vi "AI-Measure.vi"() -> ()   [LabVIEW 2016]
uses:
  <vilib>/DAQmx/read.llb/DAQmx Read (Analog Wfm 1Chan NSamp).vi
  <vilib>/DAQmx/miscellaneous.llb/DAQmx Fill In Error Info.vi
  <vilib>/Waveform/WDTFileIO.llb/Export Waveforms To Spreadsheet File (1D).vi
  <vilib>/Analysis/NI_AALBase.lvlib
  <vilib>/ptbypt/NI_PtbyPt.lvlib
panel:
  out "Signal Output":waveform(dbl)(graph)
  in  "file path (dialog if empty)":path
  out "Histogram Graph":T1(graph)
  out "Convergence of Standard Deviation":dbl[](graph)
  in  "Sample Time (s)":dbl=-1.0
  out "Convergence of Mean":dbl[](graph)
  out "standard deviation":dbl format="%0.2f"
  out "mean":dbl format="%0.2f"
  out "size(s)":i32
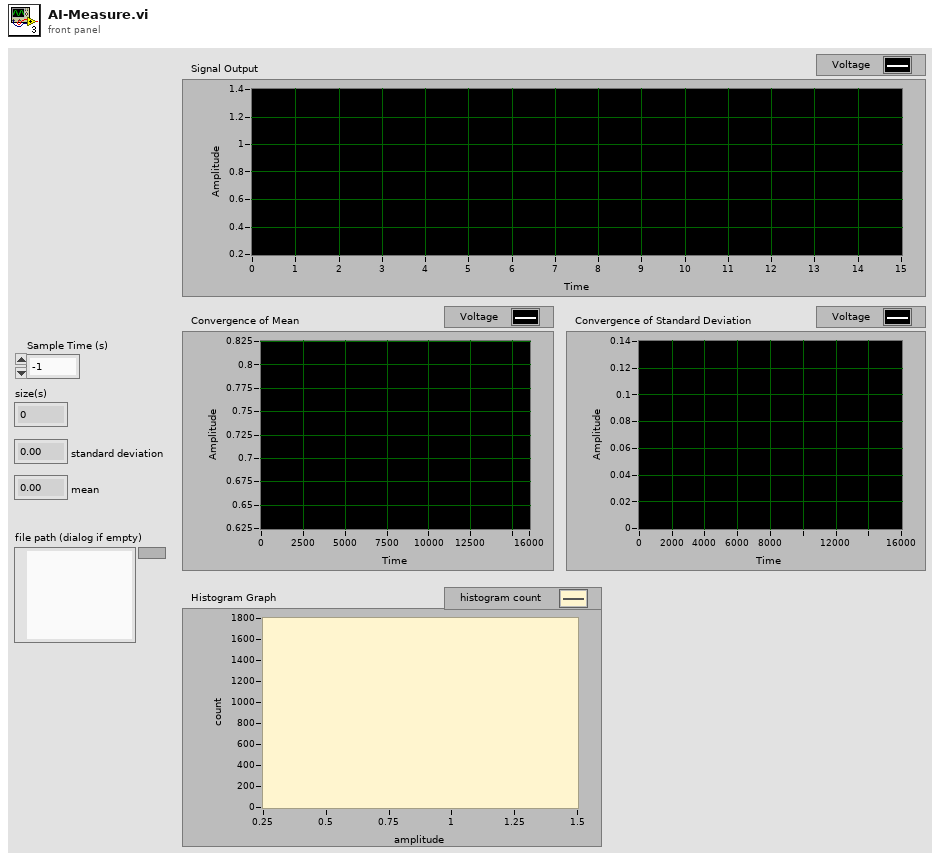
[diagram p1: front panel]
types:
  T1 = cluster{"X Values":dbl[], "Histogram: h(x)":i32[]}
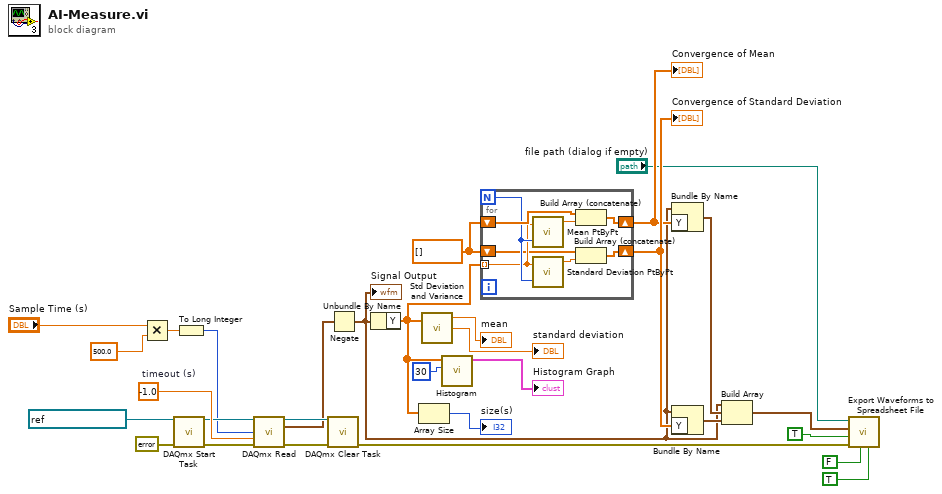
[diagram p0: block diagram]
diagram:
  w16 = dbl[] []
  w28 = -1.0  # timeout (s)
  n1 = Multiply(x="Sample Time (s)", y=500.0 ("Sample Time (s)")) -> (x*y=w18:dbl)
  n2 = call <vilib>:"DAQmx Start Task.vi"("task/channels in"=refnum<k21> "PressureVolts", "error in"=errorcluster {"status"=FALSE, "code"=0, "source"=""}) -> ("task out"=w26:refnum<k21>, "error out"=w25:errorcluster)  [unwired: 12 in]
  n3 = To Long Integer(number=w18) -> (32bit integer=w17:i32)
  n4 = call-poly <vilib>:"DAQmx Read.vi"("task/channels in"=w26, "number of samples per channel"=w17, "timeout"=w28, "error in"=w25) -> ("task out"=w30:refnum<k21>, "data"=w2:waveform(dbl), "error out"=w29:errorcluster)  [unwired: 9 in]
  n5 = call <vilib>:"DAQmx Clear Task.vi"("task in"=w30, "error in"=w29) -> ("error out"=w12:errorcluster)  [unwired: 13 in]
  n6 = Negate(x=w2) -> (-x=w1:waveform(dbl))
  "Signal Output" <- w1
  n7 = Unbundle By Name(w1) -> ("Y"=w6:dbl[])
  n8 = Array Size(array=w6) -> (size(s)=→"size(s)":i32)
  n9 = call <vilib>:"Std Deviation and Variance.vi"("X"=w6) -> ("mean"=→"mean":dbl, "standard deviation"=→"standard deviation":dbl)  [unwired: 1 in, 1 out]
  n10 = call <vilib>:"Histogram.vi"("intervals"=30, "X"=w6) -> ("Histogram Graph"=→"Histogram Graph":T1)  [unwired: 6 in, 3 out]
  n11 = for {
    N -> [w35]
    tunnel: w6 -> [w34] mode=indexing
    shift-right: [w37] -> w14
    shift-left: w16 -> [w36]
    shift-right: [w31] -> w15
    shift-left: w16 -> [w32]
    n12 = call <vilib>:"Mean PtByPt.vi"("x"=w34, "sample length"=w35) -> ("mean"=w38:dbl)  [unwired: 2 in, 1 out]
    n13 = call <vilib>:"Standard Deviation PtByPt.vi"("x"=w34, "sample length"=w35) -> ("standard deviation"=w33:dbl)  [unwired: 1 in, 2 out]
    n14 = Build Array (concatenate)(w36, w38) -> (w37:dbl[])
    n15 = Build Array (concatenate)(w32, w33) -> (w31:dbl[])
  }
  "Convergence of Mean" <- w14
  "Convergence of Standard Deviation" <- w15
  n16 = Bundle By Name(cluster=w1, "Y"=w14) -> (w8:waveform(dbl))
  n17 = Bundle By Name(cluster=w1, "Y"=w15) -> (w7:waveform(dbl))
  n18 = Build Array(w1, w8, w7) -> (w13:waveform(dbl)[])
  n19 = call-poly <vilib>:"Export Waveforms to Spreadsheet File.vi"("header? (write header:T)"=TRUE, "append to file? (new file:F)"=FALSE, "error in (no error)"=w12, "multiple time columns? (single:F)"=TRUE, "waveforms"=w13, "file path (dialog if empty)"="file path (dialog if empty)") -> ()  [unwired: 4 in, 2 out]
